vi "DAQmx Create Channel (AO-Current-Basic).vi"(0 "task in":refnum<k21>, 1 "maximum value":dbl=0.02 format="%0.5f", 2 "minimum value":dbl format="%0.5f", 5 "physical channels":tag, 7 "name to assign":string, 9 "units":i32(ring)=10342 items=["Amps"=10342, "From Custom Scale"=10065], 11 "error in":errorcluster, 12 "custom scale name":tag) -> (4 "task out":refnum<k21>, 15 "error out":errorcluster)   [LabVIEW 2018]
doc: "Creates channel(s) to generate current."
uses:
  nilvaiu.dll
panel:
  # "output limits"
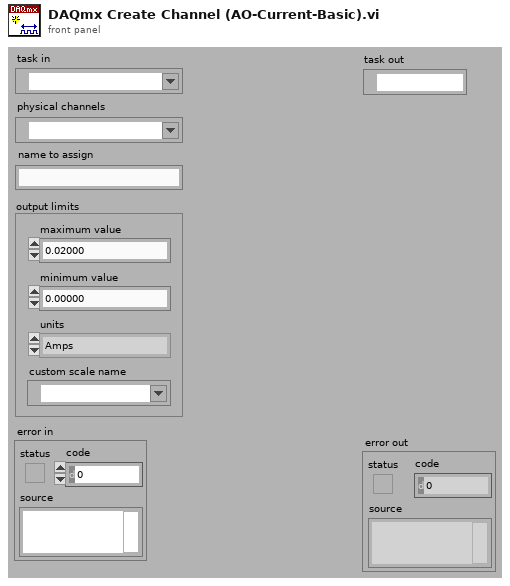
[diagram p1: front panel]
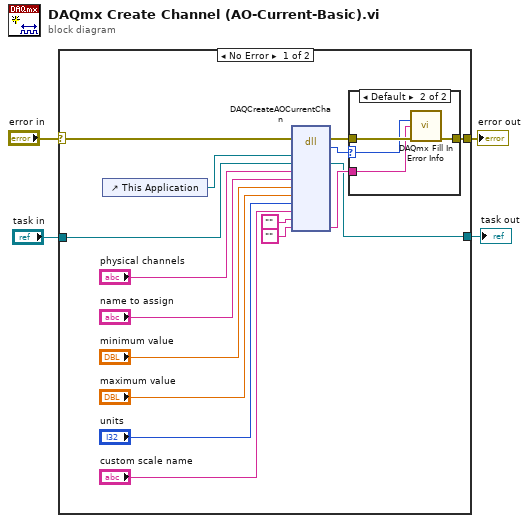
[diagram p0: block diagram]
diagram:
  n1 = case shown="No Error" "error in" {
    selector: "error in" -> [w6 w26]
    tunnel: [w15 w26] -> w4
    tunnel: [w14 w27] -> w3
    tunnel: "task in" -> [w13 w27]
    frame No Error {
      n2 = control-ref of="This Application"() -> (w20:refnum<vi>)
      n3 = dll-call lib="nilvaiu.*" fn="DAQCreateAOCurrentChan"(error in=w6, "lvAppRef"=w20, "refObjPtr"=w13, "physicalChannelName"="physical channels", "channelNameIn"="name to assign", "minVal"="minimum value", "maxVal"="maximum value", "units"="units", "customScaleName"="custom scale name", "channelNamesOut"="", "extendedErrorInfo"="") -> (error out=w16:errorcluster, "return type"=w18:i32, "refObjPtr"=w14:refnum<k21>, "extendedErrorInfo"=w19:string)  [unwired: 10 in, 1 out]
      n4 = case shown="Default" w18 {
        selector: w18 -> [_ w23]
        tunnel: w16 -> [w21 w25]
        tunnel: [w21 w24] -> w15
        tunnel: w19 -> [_ w22]
        frame 0 {
        }
        frame Default {
          n5 = call "DAQmx Fill In Error Info.vi"("status code"=w23, "extended error info"=w22, "error in"=w25) -> ("error out"=w24:errorcluster)  [unwired: 1 in, 11 out]
        }
      }
    }
    frame Error {
    }
  }
  "error out" <- w4
  "task out" <- w3
